vi "main.vi"() -> ()   [LabVIEW 2018]
uses:
  <vilib>/Instr/_visa.llb/VISA Configure Serial Port (Instr).vi
panel:
  out "当前终端节点编号":i32[](array[numeric])
  out "当前连接节点数量":dbl
  in  "停止":bool
  in  "串口写出":string
  in  "唤醒":bool
  in  "选项卡控件":enum32{"用户管理", "参数配置", "网络监视", "数据管理", "实时显示"}(tab)
  in  "用户管理":bool
  in  "修改密码":bool
  in  "登录":bool
  in  "密码":string
  in  "用户名":string
  in  "电池电量报警阈值":dbl(slide)=20.252525252525253 min=0.0 max=100.0 scale=0.0..100.0 scale format="%d%%"
  in  "设计位移":dbl[](array[numeric])
  in  "设计载荷":dbl[](array[numeric])
  in  "位移报警阈值":dbl=10.0
  in  "数据位数":dbl=8.0
  in  "波特率":dbl=9600.0
  in  "终端节点数量":dbl=200.0
  in  "汇聚节点数量":dbl=15.0
  in  "串口号":refnum<visa-resource-name>="COM1" caption="选择串口"
  in  "采样间隔":dbl
  in  "载荷报警阈值":dbl=10.0
  out "终端节点 181-200":bool[](array[boolean])
  out "终端节点 161-180":bool[](array[boolean])
  out "终端节点 141-160":bool[](array[boolean])
  out "终端节点 121-140":bool[](array[boolean])
  out "终端节点 101-120":bool[](array[boolean])
  out "终端节点 081-100":bool[](array[boolean])
  out "终端节点 061-080":bool[](array[boolean])
  out "终端节点 041-060":bool[](array[boolean])
  out "终端节点 021-040":bool[](array[boolean])
  out "协调器":bool
  out "汇聚节点":bool[](array[boolean])
  out "终端节点 001-020":bool[](array[boolean])
  out "编号":dbl
  in  "结束时间":timestamp=timestamp(3681096774.9543056 s since 1904-01-01) format="%<%Y/%m/%d %H:%M:%S>T"
  in  "打印":bool
  in  "查询按钮":bool
  out "位移":dbl[](graph)
  in  "回放吊点号":string="1"
  in  "起始时间":timestamp=timestamp(3649474370.143432 s since 1904-01-01) format="%<%Y/%m/%d %H:%M:%S>T"
  out "载荷":dbl[](graph)
  in  "选项卡控件 2":T1(tab)
  in  "选择 5":bool[](array[boolean])=[FALSE, FALSE, FALSE, FALSE, FALSE, FALSE, FALSE, FALSE, FALSE, FALSE, FALSE, FALSE, FALSE, FALSE, FALSE, FALSE, FALSE, FALSE, FALSE, FALSE, FALSE, FALSE, FALSE, FALSE, FALSE, FALSE, FALSE, FALSE, FALSE, FALSE, FALSE, FALSE, FALSE, FALSE, FALSE, FALSE, FALSE, FALSE, FALSE, FALSE]
  in  "选择 4":bool[](array[boolean])=[FALSE, FALSE, FALSE, FALSE, FALSE, FALSE, FALSE, FALSE, FALSE, FALSE, FALSE, FALSE, FALSE, FALSE, FALSE, FALSE, FALSE, FALSE, FALSE, FALSE, FALSE, FALSE, FALSE, FALSE, FALSE, FALSE, FALSE, FALSE, FALSE, FALSE, FALSE, FALSE, FALSE, FALSE, FALSE, FALSE, FALSE, FALSE, FALSE, FALSE]
  in  "选择 3":bool[](array[boolean])=[FALSE, FALSE, FALSE, FALSE, FALSE, FALSE, FALSE, FALSE, FALSE, FALSE, FALSE, FALSE, FALSE, FALSE, FALSE, FALSE, FALSE, FALSE, FALSE, FALSE, FALSE, FALSE, FALSE, FALSE, FALSE, FALSE, FALSE, FALSE, FALSE, FALSE, FALSE, FALSE, FALSE, FALSE, FALSE, FALSE, FALSE, FALSE, FALSE, FALSE]
  in  "选择 2":bool[](array[boolean])=[FALSE, FALSE, FALSE, FALSE, FALSE, FALSE, FALSE, FALSE, FALSE, FALSE, FALSE, FALSE, FALSE, FALSE, FALSE, FALSE, FALSE, FALSE, FALSE, FALSE, FALSE, FALSE, FALSE, FALSE, FALSE, FALSE, FALSE, FALSE, FALSE, FALSE, FALSE, FALSE, FALSE, FALSE, FALSE, FALSE, FALSE, FALSE, FALSE, FALSE]
  out "编号":dbl[](array[numeric])
  out "载荷":dbl[](array[numeric])
  out "位移":dbl[](array[numeric])
  out "设计载荷":dbl[](array[numeric])
  out "设计位移":dbl[](array[numeric])
  out "电池电量":bool[](array[boolean])
  out "警报":bool[](array[boolean])
  in  "选择":bool[](array[boolean])=[FALSE, FALSE, FALSE, FALSE, FALSE, FALSE, FALSE, FALSE, FALSE, FALSE, FALSE, FALSE, FALSE, FALSE, FALSE, FALSE, FALSE, FALSE, FALSE, FALSE, FALSE, FALSE, FALSE, FALSE, FALSE, FALSE, FALSE, FALSE, FALSE, FALSE, FALSE, FALSE, FALSE, FALSE, FALSE, FALSE, FALSE, FALSE, FALSE, FALSE]
  out "吊点号":string[](array[string])
  out "警报01-20":bool[](array[boolean])
  out "电池电量01-20":bool[](array[boolean])
  out "设计位移01-20":dbl[](array[numeric])
  out "设计载荷01-20":dbl[](array[numeric])
  out "位移01-20":dbl[](array[numeric])
  out "载荷01-20":dbl[](array[numeric])
  out "编号01-20":dbl[](array[numeric])
  out "吊点号01-20":string[](array[string])
  out "编号21-40":dbl[](array[numeric])
  out "载荷21-40":dbl[](array[numeric])
  out "位移21-40":dbl[](array[numeric])
  out "设计载荷21-40":dbl[](array[numeric])
  out "设计位移21-40":dbl[](array[numeric])
  out "电池电量21-40":bool[](array[boolean])
  out "警报21-40":bool[](array[boolean])
  out "吊点号21-40":string[](array[string])
  out "编号41-60":dbl[](array[numeric])
  out "载荷41-60":dbl[](array[numeric])
  out "位移41-60":dbl[](array[numeric])
  out "设计载荷41-60":dbl[](array[numeric])
  out "设计位移41-60":dbl[](array[numeric])
  out "电池电量41-60":bool[](array[boolean])
  out "警报41-60":bool[](array[boolean])
  out "吊点号41-60":string[](array[string])
  out "编号61-80":dbl[](array[numeric])
  out "载荷61-80":dbl[](array[numeric])
  out "位移61-80":dbl[](array[numeric])
  out "设计载荷61-80":dbl[](array[numeric])
  out "设计位移61-80":dbl[](array[numeric])
  out "电池电量61-80":bool[](array[boolean])
  out "警报61-80":bool[](array[boolean])
  out "吊点号61-80":string[](array[string])
  out "编号81-100":dbl[](array[numeric])
  out "载荷81-100":dbl[](array[numeric])
  out "位移81-100":dbl[](array[numeric])
  out "设计载荷81-100":dbl[](array[numeric])
  out "设计位移81-100":dbl[](array[numeric])
  out "电池电量81-100":bool[](array[boolean])
  out "警报81-100":bool[](array[boolean])
  out "吊点号81-100":string[](array[string])
  out "编号101-120":dbl[](array[numeric])
  out "载荷101-120":dbl[](array[numeric])
  out "位移101-120":dbl[](array[numeric])
  out "设计载荷101-120":dbl[](array[numeric])
  out "设计位移101-120":dbl[](array[numeric])
  out "电池电量101-120":bool[](array[boolean])
  out "警报101-120":bool[](array[boolean])
  out "吊点号101-120":string[](array[string])
  out "编号121-140":dbl[](array[numeric])
  out "载荷121-140":dbl[](array[numeric])
  out "位移121-140":dbl[](array[numeric])
  out "设计载荷121-140":dbl[](array[numeric])
  out "设计位移121-140":dbl[](array[numeric])
  out "电池电量121-140":bool[](array[boolean])
  out "警报121-140":bool[](array[boolean])
  out "吊点号121-140":string[](array[string])
  out "编号141-160":dbl[](array[numeric])
  out "载荷141-160":dbl[](array[numeric])
  out "位移141-160":dbl[](array[numeric])
  out "设计载荷141-160":dbl[](array[numeric])
  out "设计位移141-160":dbl[](array[numeric])
  out "电池电量141-160":bool[](array[boolean])
  out "警报141-160":bool[](array[boolean])
  out "吊点号141-160":string[](array[string])
  out "编号161-180":dbl[](array[numeric])
  out "载荷161-180":dbl[](array[numeric])
  out "位移161-180":dbl[](array[numeric])
  out "设计载荷161-180":dbl[](array[numeric])
  out "设计位移161-180":dbl[](array[numeric])
  out "电池电量161-180":bool[](array[boolean])
  out "警报161-180":bool[](array[boolean])
  out "吊点号161-180":string[](array[string])
  out "编号181-200":dbl[](array[numeric])
  out "载荷181-200":dbl[](array[numeric])
  out "位移181-200":dbl[](array[numeric])
  out "设计载荷181-200":dbl[](array[numeric])
  out "设计位移181-200":dbl[](array[numeric])
  out "电池电量181-200":bool[](array[boolean])
  out "警报181-200":bool[](array[boolean])
  out "吊点号181-200":string[](array[string])
  out "更新数据时间":timestamp format="%<%Y/%m/%d %H:%M:%S>T"
  in  "采集":bool
  # "C#01%001F1.11S2.11P0.11%%002F1.12S2.12P0.22%%003F1.13S2.13P0.33%%004F1.14S2.14P0.44%%005F1.15S2.15P0.55%##02%006F1.11S2.11P0.11%%007F1.12S2.12P0.22%%008F1.13S2.13P0.33%%009F1.14S2.14P0.44%%010F1.15S2.15P0.55%#C"
  # "恒力弹簧支吊架状态自动监测系统"
  # "终\n端\n0\n0\n1\n|\n0\n2\n0"
  # "终\n端\n0\n2\n1\n|\n0\n4\n0"
  # "终\n端\n0\n4\n1\n|\n0\n6\n0"
  # "终\n端\n0\n6\n1\n|\n0\n8\n0"
  # "终\n端\n0\n8\n1\n|\n1\n0\n0"
  # "终\n端\n1\n0\n1\n|\n1\n2\n0"
  # "终\n端\n1\n2\n1\n|\n1\n4\n0"
  # "终\n端\n1\n4\n1\n|\n1\n6\n0"
  # "终\n端\n1\n6\n1\n|\n1\n8\n0"
  # "终\n端\n1\n8\n1\n|\n2\n0\n0"
  # "0          0          0          1          1  \n0          4          8          2          6\n1          1          1          1          1\n|           |           |           |           |\n0          0          1          1          2\n4          8          2          6          0\n0          0          0          0          0"
  # "编号               吊点号              载荷                 位移                警报             电池电量          设计载荷           设计位移"
  # "编号                   吊点号                 载荷                  位移                  警报               电池电量            设计载荷           设计位移"
  # "编号                   吊点号                 载荷                  位移                  警报               电池电量            设计载荷           设计位移"
  # "编号                   吊点号                 载荷                  位移                  警报               电池电量            设计载荷           设计位移"
  # "编号                   吊点号                 载荷                  位移                  警报               电池电量            设计载荷           设计位移"
  # "编号                   吊点号                 载荷                  位移                  警报               电池电量            设计载荷           设计位移"
  # "编号                   吊点号                 载荷                  位移                  警报               电池电量            设计载荷           设计位移"
  # "编号                   吊点号                 载荷                  位移                  警报               电池电量            设计载荷           设计位移"
  # "编号                   吊点号                 载荷                  位移                  警报               电池电量            设计载荷           设计位移"
  # "编号                   吊点号                 载荷                  位移                  警报               电池电量            设计载荷           设计位移"
  # "编号                   吊点号                 载荷                  位移                  警报               电池电量            设计载荷           设计位移"
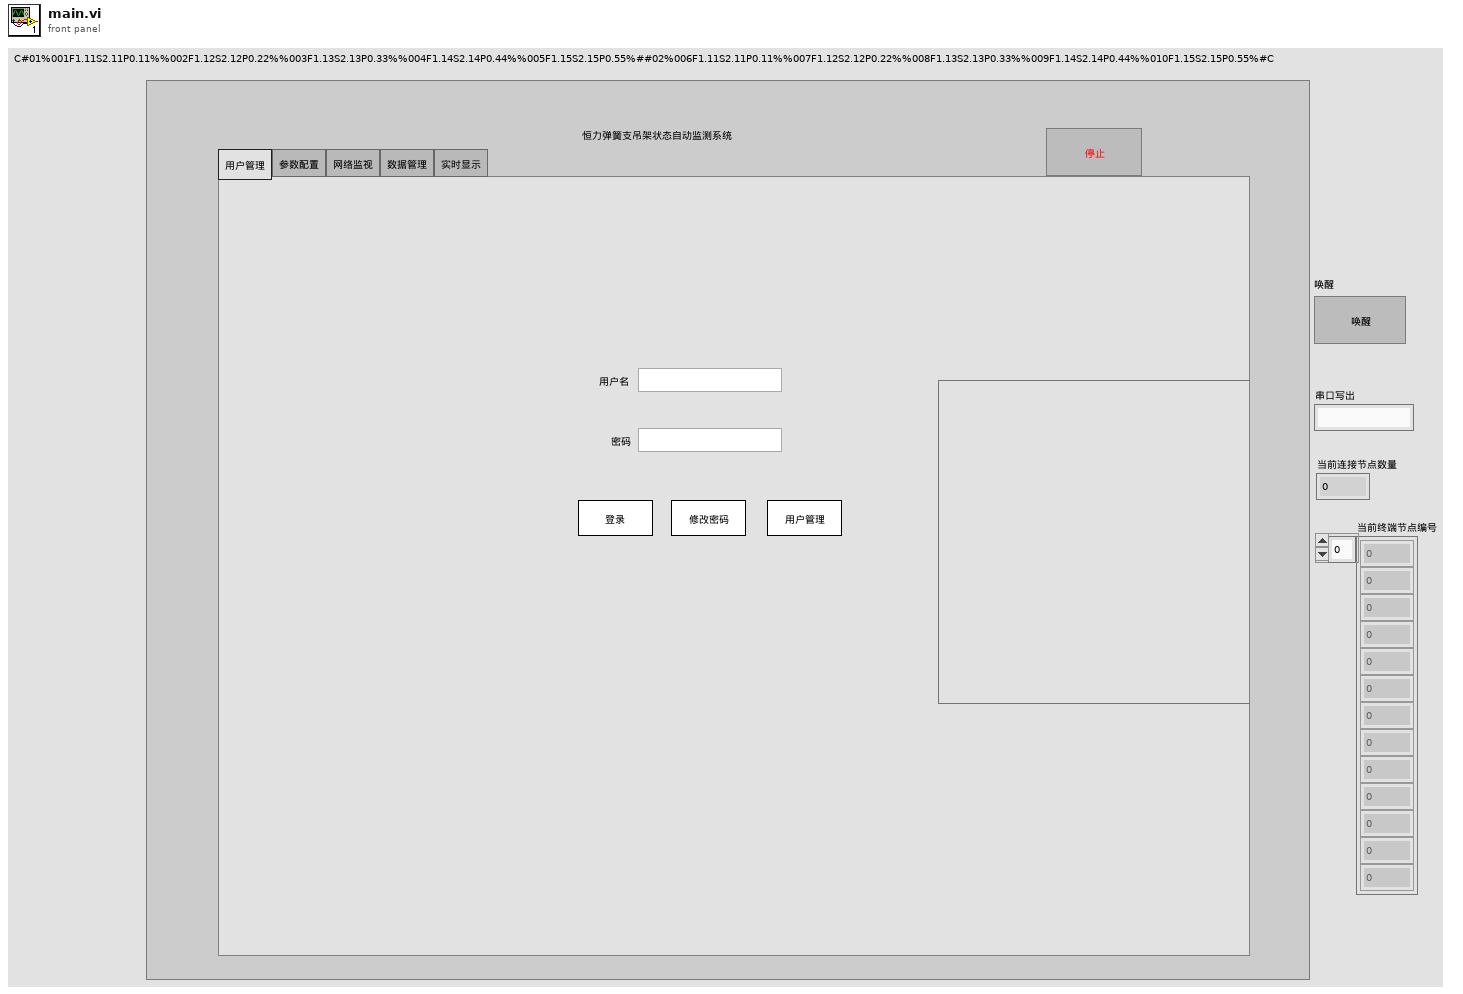
[diagram p1: front panel]
types:
  T1 = enum32{"请选择20个", "001-020", "021-040", "041-060", "061-080", "081-100", "101-120", "121-140", "141-160", "161-180", "181-200"}
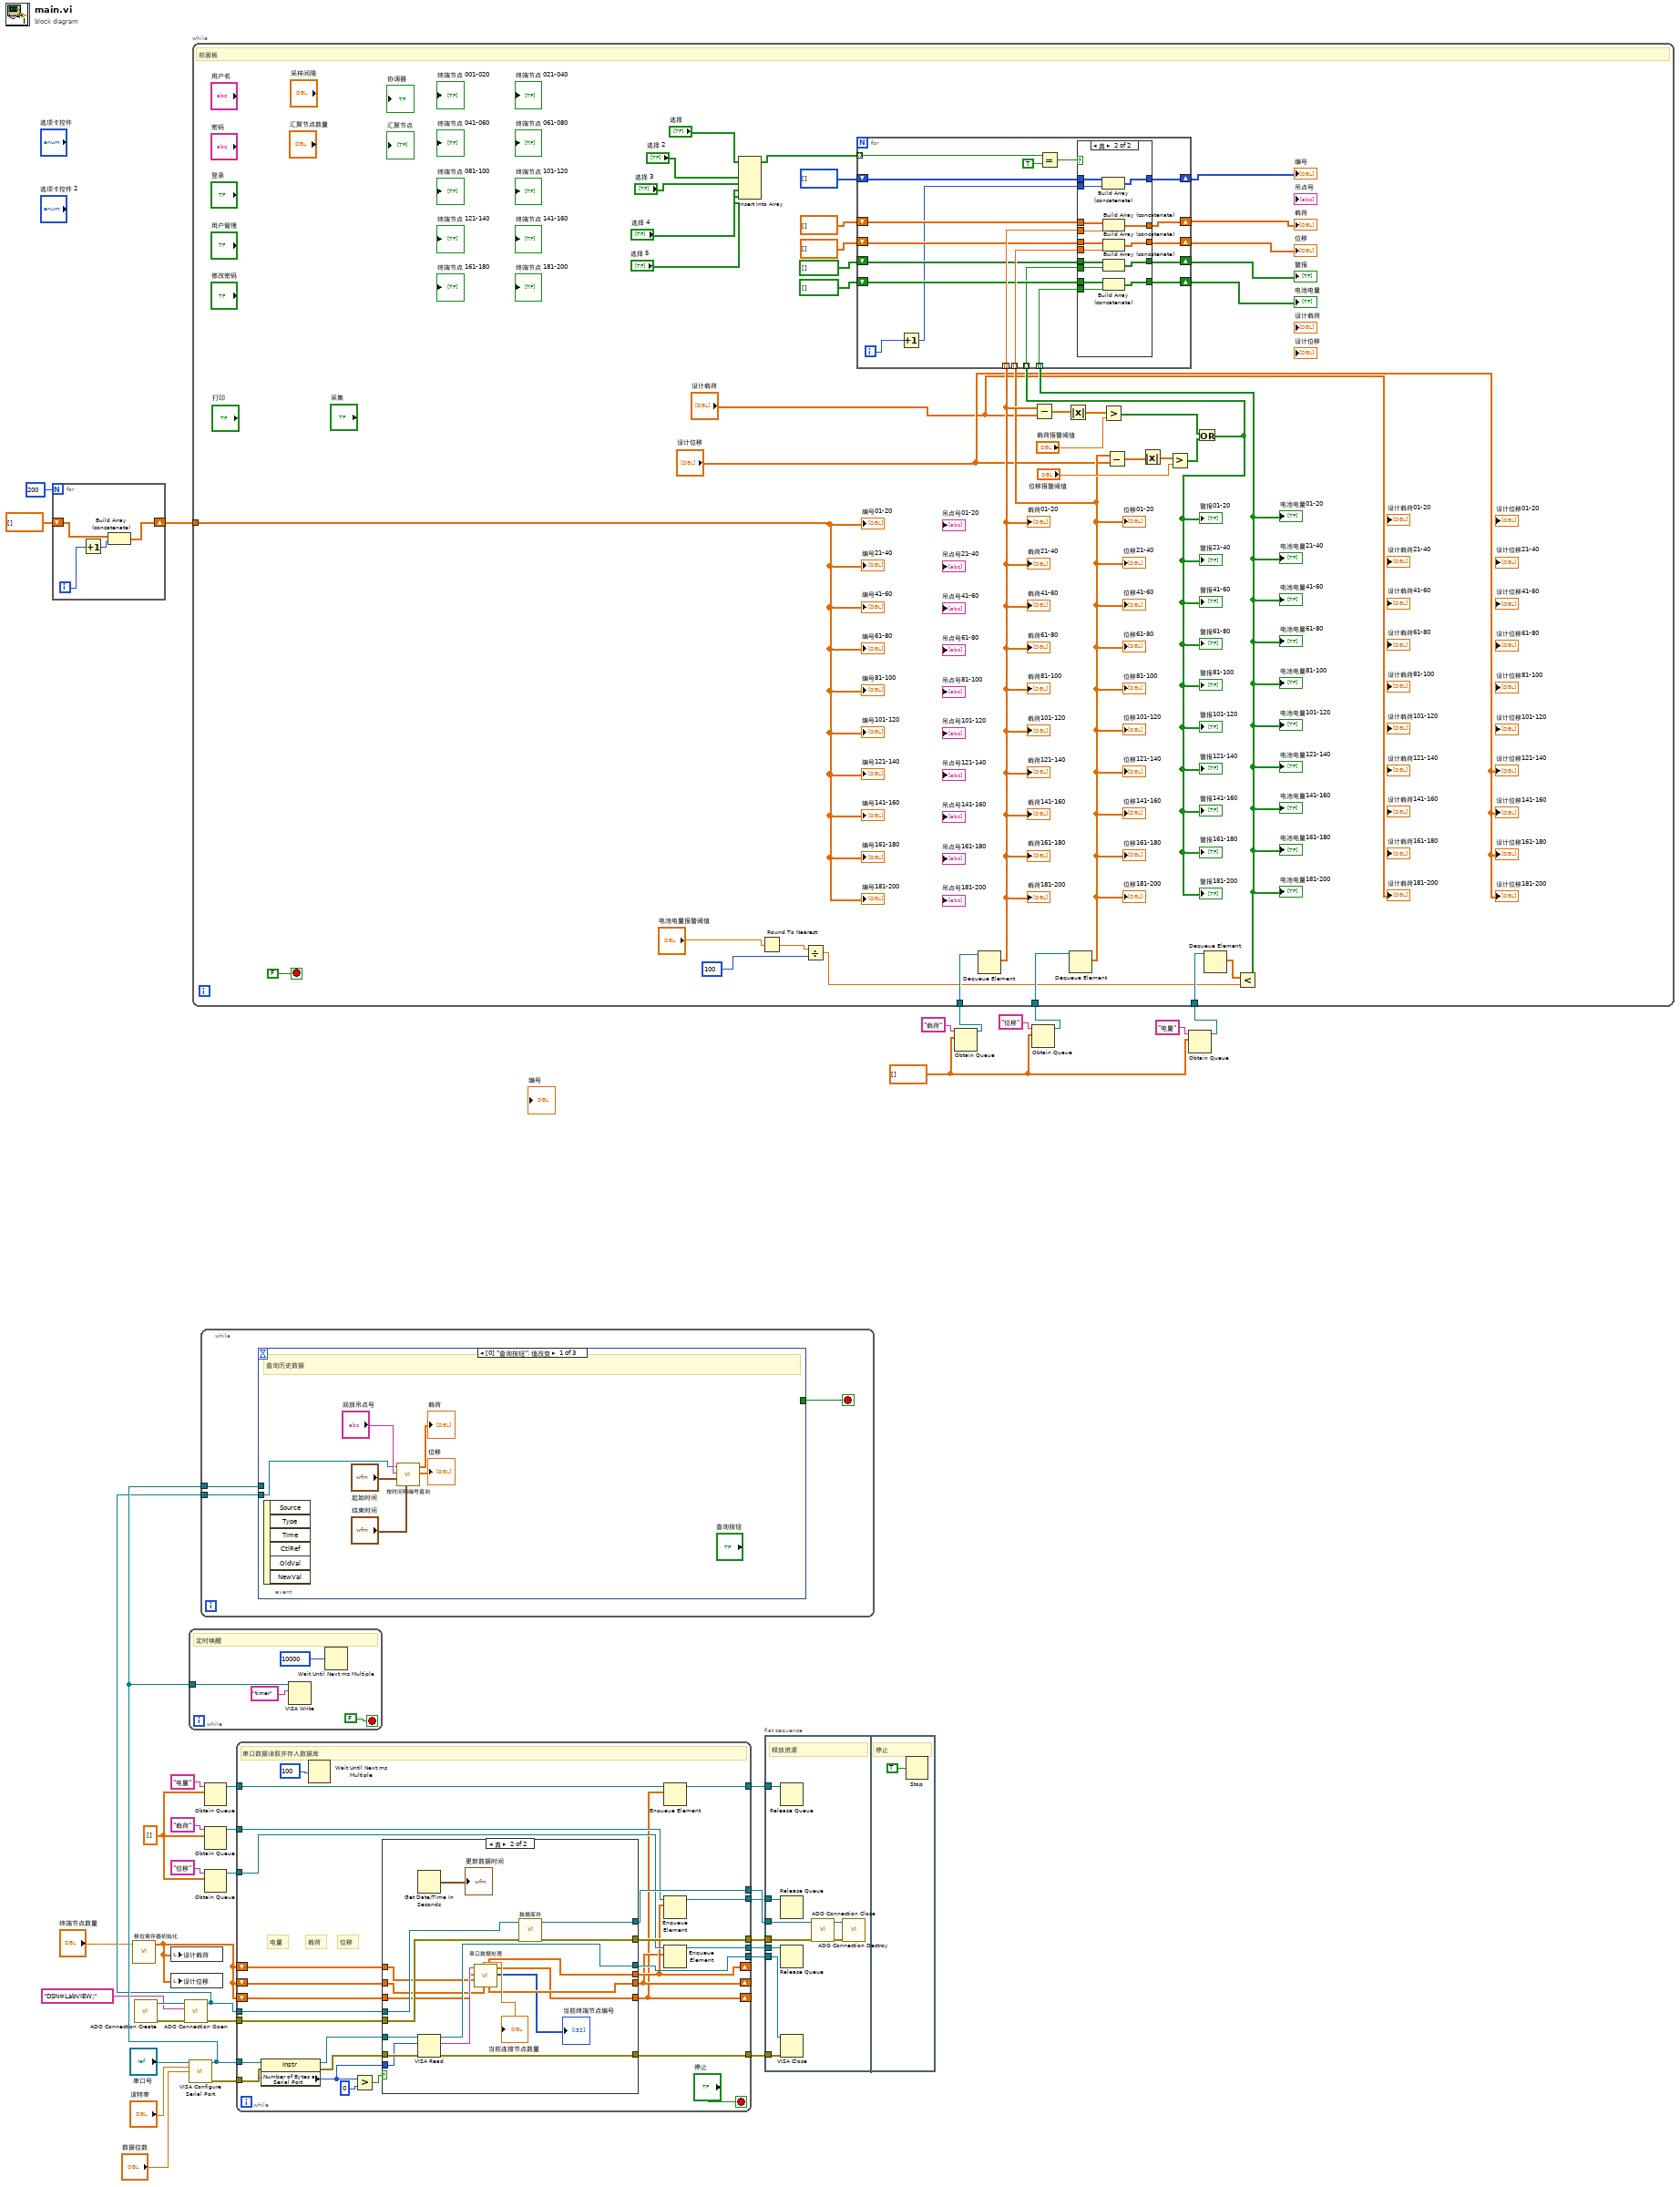
[diagram p0: block diagram]
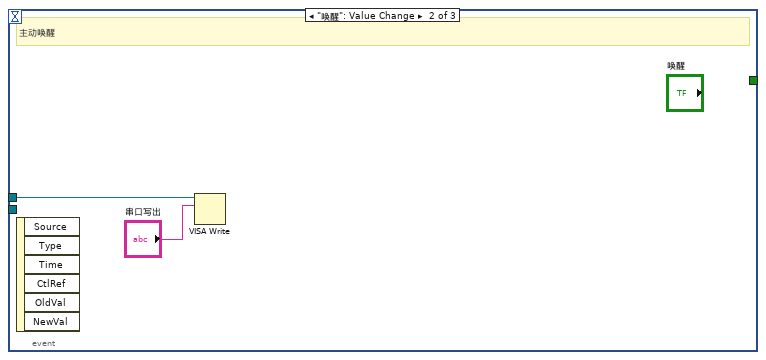
[diagram p3: hidden frame]
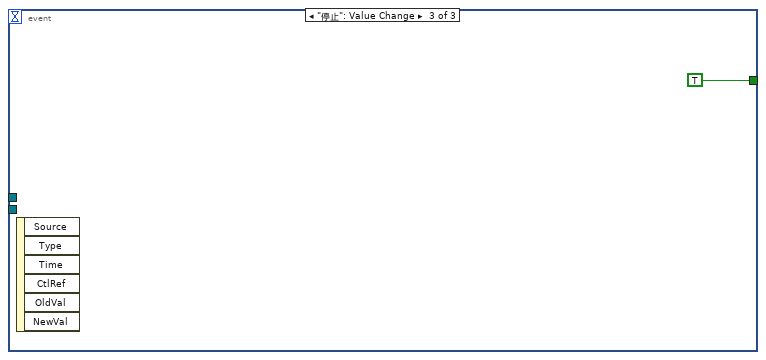
[diagram p4: hidden frame]
diagram:
  w9 = dbl[] []
  w30 = dbl[] []
  n1 = for {
    N: 200 -> [_]
    shift-right: [w39] -> w5
    shift-left: dbl[] [] -> [w40]
    i -> [w38]
    n2 = Increment(x=w38) -> (x+1=w37:i32)
    n3 = Build Array (concatenate)(w40, w37) -> (w39:dbl[])
  }
  n4 = call "移位寄存器初始化.vi"("终端节点数量"="终端节点数量") -> ("数组"=w1:dbl[])  [unwired: 10 in]
  n5 = call <userlib>:"ADO Connection Create.vi"() -> ("error out"=w21:errorcluster, "ADODB._Connection Out"=w22:refnum<k7>)  [unwired: 10 in]
  n6 = local write "设计载荷"(w1) -> ()
  n7 = local write "设计位移"(w1) -> ()
  n8 = call <userlib>:"ADO Connection Open.vi"("error in (no error)"=w21, "ConnectionString"="DSN=LabVIEW;", "ADODB._Connection In"=w22) -> ("error out"=w23:errorcluster, "ADODB._Connection Out"=w19:refnum<k7>)  [unwired: 7 in]
  n9 = call-poly "VISA Configure Serial Port"("VISA resource name"="串口号", "baud rate (9600)"="波特率", "data bits (8)"="数据位数") -> ("VISA resource name out"=w26:refnum<visa-resource-name>, "error out"=w28:errorcluster)  [unwired: 11 in]
  n10 = while {
    tunnel: w26 -> [w43]
    stop <- FALSE stop-if-true
    # "定时唤醒"
    n11 = VISA Write(VISA resource name=w43, write buffer="timer" ("写入缓冲区")) -> ()  [unwired: 1 in, 3 out]
    n12 = Wait Until Next ms Multiple(millisecond multiple=u32 10000 ("毫秒倍数")) -> ()  [unwired: 1 out]
  }
  n13 = while {
    tunnel: w26 -> [w46]
    tunnel: w19 -> [w45]
    stop <- w47 stop-if-true
    n14 = event shown="[0] \"查询按钮\": 值改变" {
      selector: _ -> [_ _ _]
      dyn-events: _ -> [_ _ _]
      timeout: _ -> [_ _ _]
      tunnel: [_ _ TRUE] -> w47
      tunnel: w46 -> [_ w54 _]
      tunnel: w45 -> [w52 _ _]
      event "查询按钮": Value Change {
        # "查询历史数据"
        n15 = event-data() -> ()  [unwired: 1 in, 6 out]
        n16 = call "按时间和编号查询.vi"("结束时间"="结束时间", "起始时间"="起始时间", "回放吊点号"="回放吊点号", "自动化引用句柄输入"=w52) -> ("位移"=→"位移":dbl[], "载荷"=→"载荷":dbl[])  [unwired: 6 in]
      }
      event "唤醒": Value Change {
        # "主动唤醒"
        n17 = event-data() -> ()  [unwired: 1 in, 6 out]
        n18 = VISA Write(VISA resource name=w54, write buffer="串口写出") -> ()  [unwired: 1 in, 3 out]
      }
      event "停止": Value Change {
        n19 = event-data() -> ()  [unwired: 1 in, 6 out]
      }
    }
  }
  n20 = Obtain Queue(name (unnamed)="电量" ("写入缓冲区"), element data type=w9) -> (queue out=w11:refnum<queue>)  [unwired: 3 in, 2 out]
  n21 = Obtain Queue(name (unnamed)="载荷" ("写入缓冲区"), element data type=w9) -> (queue out=w15:refnum<queue>)  [unwired: 3 in, 2 out]
  n22 = Obtain Queue(name (unnamed)="位移" ("写入缓冲区"), element data type=w9) -> (queue out=w13:refnum<queue>)  [unwired: 3 in, 2 out]
  n23 = while "While循环" {
    tunnel: w26 -> [w79]
    tunnel: [w76] -> w29
    tunnel: w28 -> [w83]
    tunnel: [w75] -> w27
    tunnel: [w72] -> w25
    tunnel: [w71] -> w24
    tunnel: w19 -> [w70]
    tunnel: w23 -> [w69]
    shift-right: [w57] -> _
    shift-left: w1 -> [w67]
    shift-right: [w58] -> _
    shift-left: w1 -> [w68]
    shift-right: [w59] -> _
    shift-left: w1 -> [w66]
    tunnel: [w65] -> w18
    tunnel: [w64] -> w17
    tunnel: w15 -> [w63]
    tunnel: w13 -> [w62]
    tunnel: w11 -> [w61]
    tunnel: [w60] -> w10
    stop <- "停止" stop-if-true
    # "电量"
    # "位移"
    # "载荷"
    # "串口数据读取并存入数据库"
    n24 = property class="Instr"(reference=w79, error in=w83) -> (reference out=w73:refnum<visa-resource-name>, error out=w74:errorcluster, "Serial Settings:Number of Bytes at Serial Port"=w80:u32)
    n25 = Wait Until Next ms Multiple(millisecond multiple=u32 100 ("毫秒倍数")) -> ()  [unwired: 1 out]
    n26 = Greater?(x=w80, y=u32 0) -> (0:w81:bool)
    n27 = case shown="真" w81 {
      tunnel: w73 -> [w90 w109]
      tunnel: [w90 w105] -> w76
      tunnel: w74 -> [w89 w108]
      tunnel: [w89 w106] -> w75
      tunnel: w80 -> [_ w107]
      tunnel: [w87 w104] -> w72
      tunnel: [w88 w103] -> w71
      tunnel: w70 -> [w87 w102]
      tunnel: w69 -> [w88 w101]
      tunnel: [w86 w93] -> w58
      tunnel: [w84 w94] -> w59
      tunnel: [w85 w92] -> w57
      tunnel: w68 -> [w86 w96]
      tunnel: w67 -> [w85 w98]
      tunnel: w66 -> [w84 w97]
      frame False {
      }
      frame True {
        n28 = Get Date/Time In Seconds() -> (seconds since 1Jan1904=→"更新数据时间":timestamp)
        n29 = VISA Read(VISA resource name=w109, byte count=w107, error in (no error)=w108) -> (VISA resource name out=w105:refnum<visa-resource-name>, read buffer=w99:string, error out=w106:errorcluster)  [unwired: 1 out]
        n30 = call "串口数据处理.vi"("位移输入"=w96, "载荷输入"=w97, "电量输入"=w98, "read buffer"=w99) -> ("当前终端节点编号"=→"当前终端节点编号":i32[], "电量输出"=w92:dbl[], "位移输出"=w93:dbl[], "载荷输出"=w94:dbl[], "当前连接终端节点数量"=→"当前连接节点数量":dbl)  [unwired: 2 in, 1 out]
        n31 = call "数据库存.vi"("错误输入（无错误）"=w101, "自动化引用句柄输入"=w102) -> ("错误输出"=w103:errorcluster, "自动化引用句柄输出"=w104:refnum<k7>)  [unwired: 8 in]
      }
    }
    n32 = Enqueue Element(queue=w61, element=w57) -> (queue out=w60:refnum<queue>)  [unwired: 2 in, 2 out]
    n33 = Enqueue Element(queue=w63, element=w59) -> (queue out=w65:refnum<queue>)  [unwired: 2 in, 2 out]
    n34 = Enqueue Element(queue=w62, element=w58) -> (queue out=w64:refnum<queue>)  [unwired: 2 in, 2 out]
  }
  n35 = flat-sequence {
    tunnel: w29 -> [w118]
    tunnel: w27 -> [w117]
    tunnel: w25 -> [w114]
    tunnel: w24 -> [w113]
    tunnel: w18 -> [w112]
    tunnel: w17 -> [w111]
    tunnel: w10 -> [w110]
    frame #0 {
      # "释放资源"
      n36 = Release Queue(queue=w110) -> ()  [unwired: 2 in, 3 out]
      n37 = Release Queue(queue=w112) -> ()  [unwired: 2 in, 3 out]
      n38 = Release Queue(queue=w111) -> ()  [unwired: 2 in, 3 out]
      n39 = VISA Close(VISA resource name=w118, error in (no error)=w117) -> ()  [unwired: 1 out]
      n40 = call <userlib>:"ADO Connection Close.vi"("error in (no error)"=w113, "ADODB._Connection In"=w114) -> ("error out"=w115:errorcluster, "ADODB._Connection Out"=w116:refnum<k7>)  [unwired: 8 in]
      n41 = call <userlib>:"ADO Connection Destroy.vi"("error in (no error)"=w115, "ADODB._Connection In"=w116) -> ()  [unwired: 9 in, 1 out]
    }
    frame #1 {
      # "停止"
      n42 = Stop(stop? (T)=TRUE ("停止？(T)")) -> ()
    }
  }
  n43 = Obtain Queue(name (unnamed)="载荷" ("写入缓冲区"), element data type=w30) -> (queue out=w33:refnum<queue>)  [unwired: 3 in, 2 out]
  n44 = Obtain Queue(name (unnamed)="位移" ("写入缓冲区"), element data type=w30) -> (queue out=w32:refnum<queue>)  [unwired: 3 in, 2 out]
  n45 = Obtain Queue(name (unnamed)="电量" ("写入缓冲区"), element data type=w30) -> (queue out=w31:refnum<queue>)  [unwired: 3 in, 2 out]
  n46 = while "While循环" {
    tunnel: w33 -> [w155]
    tunnel: w32 -> [w154]
    tunnel: w31 -> [w153]
    tunnel: w5 -> [w131]
    stop <- FALSE stop-if-true
    # "前面板"
    n47 = Insert Into Array(array="选择", new element #1="选择 2", new element #2="选择 3", new element #3="选择 4", new element #4="选择 5") -> (w158:bool[])  [unwired: 1 in]
    n48 = Round To Nearest(number="电池电量报警阈值") -> (nearest integer value=w123:dbl)
    n49 = Divide(x=w123, y=100) -> (x/y=w120:dbl)
    n50 = Dequeue Element(queue=w155) -> (element=w143:dbl[])  [unwired: 2 in, 3 out]
    "载荷01-20" <- w143
    "载荷21-40" <- w143
    "载荷41-60" <- w143
    "载荷61-80" <- w143
    "载荷81-100" <- w143
    "载荷101-120" <- w143
    "载荷121-140" <- w143
    "载荷141-160" <- w143
    "载荷161-180" <- w143
    "载荷181-200" <- w143
    n51 = Subtract(x=w143, y="设计载荷") -> (x-y=w151:dbl[])
    n52 = Absolute Value(x=w151) -> (abs(x)=w148:dbl[])
    n53 = Dequeue Element(queue=w154) -> (element=w140:dbl[])  [unwired: 2 in, 3 out]
    "位移01-20" <- w140
    "位移21-40" <- w140
    "位移41-60" <- w140
    "位移61-80" <- w140
    "位移81-100" <- w140
    "位移101-120" <- w140
    "位移121-140" <- w140
    "位移141-160" <- w140
    "位移161-180" <- w140
    "位移181-200" <- w140
    n54 = Greater?(x=w148, y="载荷报警阈值") -> (0:w145:bool[])
    n55 = Subtract(x=w140, y="设计位移") -> (x-y=w150:dbl[])
    n56 = Absolute Value(x=w150) -> (abs(x)=w146:dbl[])
    n57 = Greater?(x=w146, y="位移报警阈值") -> (0:w144:bool[])
    n58 = Or(x=w145, y=w144) -> (x .or. y?=w137:bool[])
    "警报01-20" <- w137
    "警报21-40" <- w137
    "警报41-60" <- w137
    "警报61-80" <- w137
    "警报81-100" <- w137
    "警报101-120" <- w137
    "警报121-140" <- w137
    "警报141-160" <- w137
    "警报161-180" <- w137
    "警报181-200" <- w137
    n59 = Dequeue Element(queue=w153) -> (element=w152:dbl[])  [unwired: 2 in, 3 out]
    n60 = Less?(x=w152, y=w120) -> (x < y?=w138:bool[])
    "电池电量01-20" <- w138
    "电池电量21-40" <- w138
    "电池电量41-60" <- w138
    "电池电量61-80" <- w138
    "电池电量81-100" <- w138
    "电池电量101-120" <- w138
    "电池电量121-140" <- w138
    "电池电量141-160" <- w138
    "电池电量161-180" <- w138
    "电池电量181-200" <- w138
    n61 = for {
      tunnel: w158 -> [w176] mode=indexing
      shift-right: [w174] -> w156
      shift-left: dbl[] [] -> [w175]
      tunnel: w143 -> [w173] mode=indexing
      shift-right: [w171] -> w141
      shift-left: dbl[] [] -> [w172]
      tunnel: w140 -> [w170] mode=indexing
      tunnel: w138 -> [w169] mode=indexing
      shift-right: [w167] -> w139
      shift-left: bool[] [] -> [w168]
      tunnel: w137 -> [w166] mode=indexing
      shift-right: [w164] -> w136
      shift-left: bool[] [] -> [w165]
      shift-right: [w162] -> w132
      shift-left: i32[] [] -> [w163]
      i -> [w161]
      n62 = Increment(x=w161) -> (x+1=w160:i32)
      n63 = Equal?(x=w176, y=TRUE) -> (x = y?=w177:bool)
      n64 = case shown="真" w177 {
        tunnel: w175 -> [w183 w198]
        tunnel: [w183 w197] -> w174
        tunnel: w173 -> [_ w196]
        tunnel: w172 -> [w182 w195]
        tunnel: [w182 w194] -> w171
        tunnel: w170 -> [_ w193]
        tunnel: w169 -> [_ w192]
        tunnel: w168 -> [w180 w191]
        tunnel: [w180 w190] -> w167
        tunnel: w166 -> [_ w189]
        tunnel: w165 -> [w181 w188]
        tunnel: [w181 w187] -> w164
        tunnel: w163 -> [w179 w186]
        tunnel: [w179 w185] -> w162
        tunnel: w160 -> [_ w184]
        frame False {
        }
        frame True {
          n65 = Build Array (concatenate)(w186, w184) -> (w185:i32[])
          n66 = Build Array (concatenate)(w198, w196) -> (w197:dbl[])
          n67 = Build Array (concatenate)(w195, w193) -> (w194:dbl[])
          n68 = Build Array (concatenate)(w188, w189) -> (w187:bool[])
          n69 = Build Array (concatenate)(w191, w192) -> (w190:bool[])
        }
      }
    }
    "编号" <- w132
    "载荷" <- w156
    "位移" <- w141
    "电池电量" <- w139
    "警报" <- w136
    "编号01-20" <- w131
    "编号21-40" <- w131
    "编号41-60" <- w131
    "编号61-80" <- w131
    "编号81-100" <- w131
    "编号101-120" <- w131
    "编号121-140" <- w131
    "设计位移121-140" <- "设计位移"
    "编号141-160" <- w131
    "设计位移141-160" <- "设计位移"
    "编号161-180" <- w131
    "设计位移161-180" <- "设计位移"
    "编号181-200" <- w131
    "设计载荷181-200" <- "设计载荷"
    "设计位移181-200" <- "设计位移"
  }
